vi "Load_waveform_multi_files.vi"(0 "Enable limit = True":bool=TRUE, 2 "Limit for Stop file#":dbl, 3 "File Limited":i8) -> (10 "File_list":path[](array[path]), 12 "Total_Duration":dbl, 14 "first waveform in record":waveform(dbl), 15 "#WF IN File":i32[](array[numeric]), 16 "selected path":path, 17 "Loop ?":i32, 18 "Duration":dbl, 19 "Sample rate":dbl)   [LabVIEW 2017]
uses:
  <vilib>/Waveform/WDTFileIO.llb/Read Waveform from File.vi
  <vilib>/Waveform/WDTOps.llb/WDT Append Waveforms DBL.vi
panel:
  out "Numeric":i32
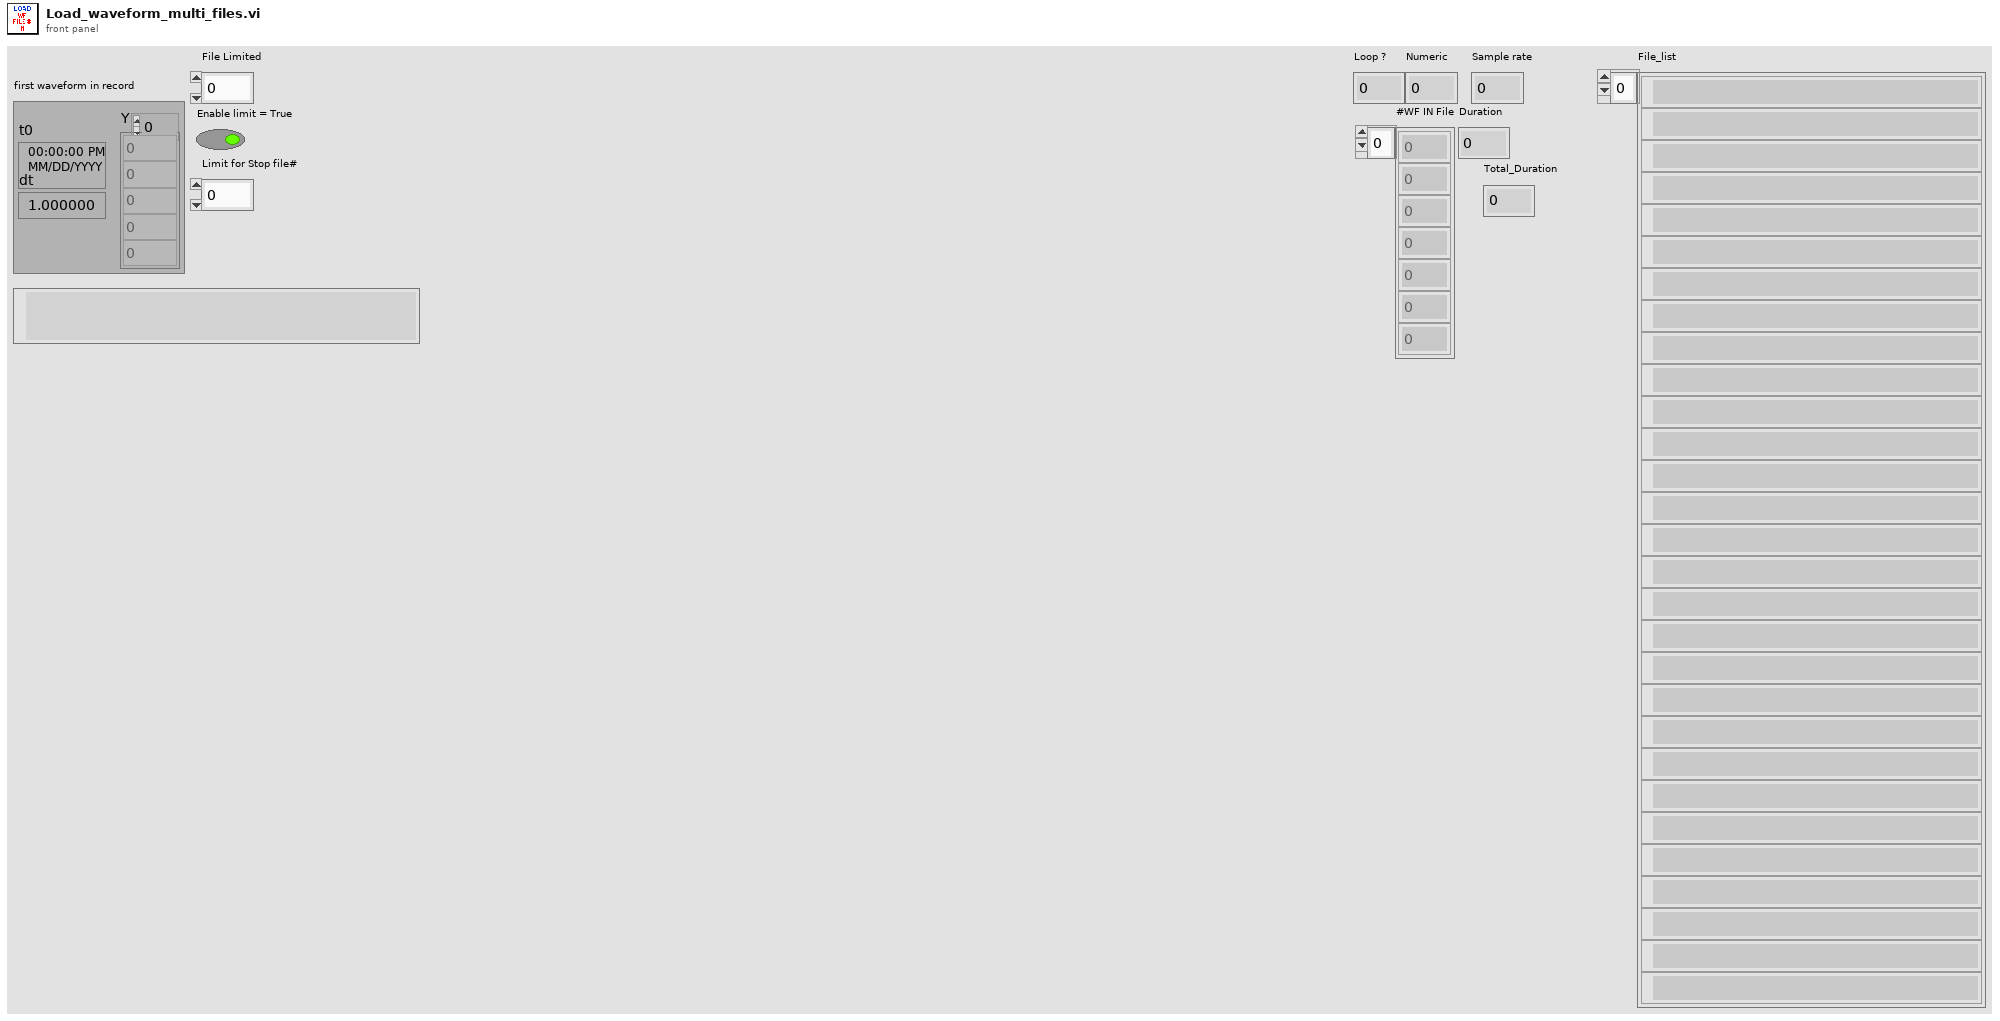
[diagram p1: front panel]
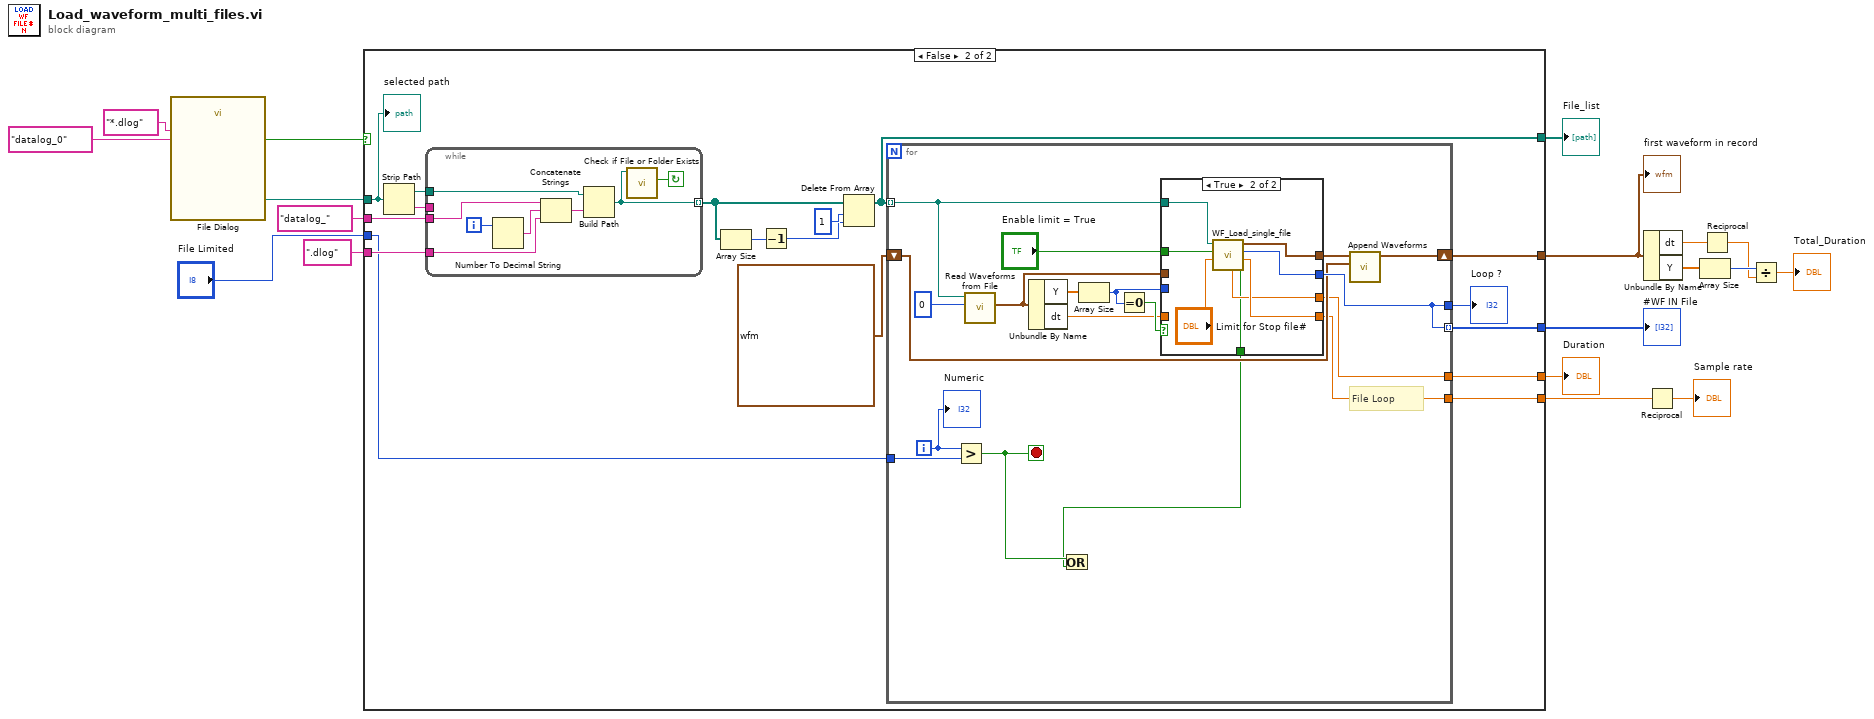
[diagram p0: block diagram]
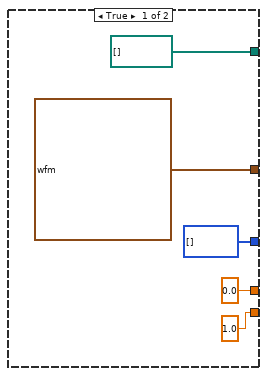
[diagram p2: hidden frame]
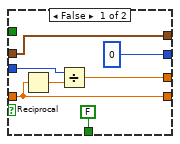
[diagram p3: hidden frame]
diagram:
  n1 = call "File Dialog"("pattern (all files)"="*.dlog", "pattern label"="datalog_0") -> ("selected path"=w16:path, "cancelled"=w15:bool)  [unwired: 10 in, 2 out]
  n2 = case shown="False" w15 {
    tunnel: w16 -> [_ w40]
    tunnel: ".dlog" ("pattern (all files)") -> [_ w37]
    tunnel: "datalog_" ("pattern label") -> [_ w36]
    tunnel: [waveform(dbl) {"t0"=timestamp(0 s since 1904-01-01), "dt"=1.0, "Y"=[]} ("waveform out") w30] -> w7
    tunnel: [1.0 ("dt") w28] -> w12
    tunnel: [path[] [] w27] -> w10
    tunnel: [0.0 w26] -> w9
    tunnel: [i32[] [] w25] -> w8
    tunnel: "File Limited" -> [_ w24]
    frame True {
    }
    frame False {
      n3 = Strip Path(path=w40) -> (stripped path=w38:path, name=w39:string)
      n4 = while {
        tunnel: w39 -> [_]
        tunnel: w38 -> [w77]
        tunnel: w37 -> [w81]
        tunnel: w36 -> [w80]
        tunnel: [w74] -> w34 mode=indexing
        i -> [w79]
        stop <- w75 continue-if-true
        n5 = Number To Decimal String(number=w79) -> (decimal integer string=w78:string)  [unwired: 1 in]
        n6 = Concatenate Strings(w80, w78, w81) -> (w76:string)
        n7 = Build Path(base path=w77, name or relative path=w76) -> (appended path=w74:path)
        n8 = call <vilib>:"Check if File or Folder Exists.vi"("path"=w74) -> ("file or folder exists?"=w75:bool)  [unwired: 8 in, 2 out]
      }
      n9 = Array Size(array=w34) -> (size(s)=w32:i32)
      n10 = Decrement(x=w32) -> (x-1=w31:i32)
      n11 = Delete From Array(array=w34, length=1, index=w31) -> (array with subset deleted=w27:path[])  [unwired: 1 out]
      n12 = for {
        tunnel: [w51] -> w35
        tunnel: w27 -> [w53] mode=indexing
        shift-right: [w52] -> w30
        shift-left: waveform(dbl) {"t0"=timestamp(0 s since 1904-01-01), "dt"=1.0, "Y"=[]} ("waveform out") -> [w50]
        tunnel: [w51] -> w25 mode=indexing
        tunnel: [w48] -> w28
        tunnel: [w46] -> w26
        tunnel: w24 -> [w43]
        i -> [w44]
        stop <- w42 stop-if-true
        # "File Loop"
        n13 = Greater?(x=w44, y=w43) -> (0:w42:bool)
        n14 = call-poly <vilib>:"Read Waveforms from File.vi"("offset (records:0)"=0, "file path (dialog if empty)"=w53) -> ("first waveform in record"=w58:waveform(dbl))  [unwired: 4 in, 3 out]
        n15 = Unbundle By Name(w58) -> ("Y"=w56:dbl[], "dt"=w47:dbl)
        n16 = Array Size(array=w56) -> (size(s)=w45:i32)
        n17 = Equal To 0?(x=w45) -> (x = 0?=w57:bool)
        n18 = case shown="True" w57 {
          tunnel: [w65 w73] -> w49
          tunnel: w53 -> [_ w72]
          tunnel: w58 -> [w65 _]
          tunnel: "Enable limit = True" -> [_ w71]
          tunnel: [0 w70] -> w51
          tunnel: [w61 w69] -> w48
          tunnel: w47 -> [w61 _]
          tunnel: [w60 w68] -> w46
          tunnel: w45 -> [w62 _]
          tunnel: [FALSE ("Stop") w66] -> w41
          frame False {
            n19 = Reciprocal(x=w61) -> (1/x=w63:dbl)
            n20 = Divide(x=w62, y=w63) -> (x/y=w60:dbl)
          }
          frame True {
            n21 = call "WF_Load_single_file.vi"("Limit for Stop file#"="Limit for Stop file#", "Enable limit = True"=w71, "WF_FILE_IN"=w72) -> ("Stop"=w66:bool, "dt"=w69:dbl, "Record#"=w70:i32, "Waveform"=w73:waveform(dbl), "File_duration(s)"=w68:dbl)  [unwired: 4 in]
          }
        }
        n22 = Or(x=w42, y=w41) -> ()  [unwired: 1 out]
        n23 = call-poly <vilib>:"Append Waveforms.vi"("waveform B"=w50, "waveform A"=w49) -> ("waveform out"=w52:waveform(dbl))  [unwired: 8 in, 1 out]
        "Numeric" <- w44
      }
      "Loop ?" <- w35
      "selected path" <- w40
    }
  }
  "first waveform in record" <- w7
  "File_list" <- w10
  "Duration" <- w9
  "#WF IN File" <- w8
  n24 = Unbundle By Name(w7) -> ("dt"=w6:dbl, "Y"=w5:dbl[])
  n25 = Reciprocal(x=w12) -> (1/x=→"Sample rate":dbl)
  n26 = Array Size(array=w5) -> (size(s)=w4:i32)
  n27 = Reciprocal(x=w6) -> (1/x=w3:dbl)
  n28 = Divide(x=w4, y=w3) -> (x/y=→"Total_Duration":dbl)
